vi "Controller.vi"   [LabVIEW 2023]
uses:
  Pulpit/GV_TakePhoto.vi
  GV_exit.vi
  GV_StartStop.vi
  GV_obraz.vi
types:
  T1 = enum16{"Standard", "Buffered", "CRLF", "Immediate"}
  T2 = typedef "IMAQ Image.ctl" = refnum<image>
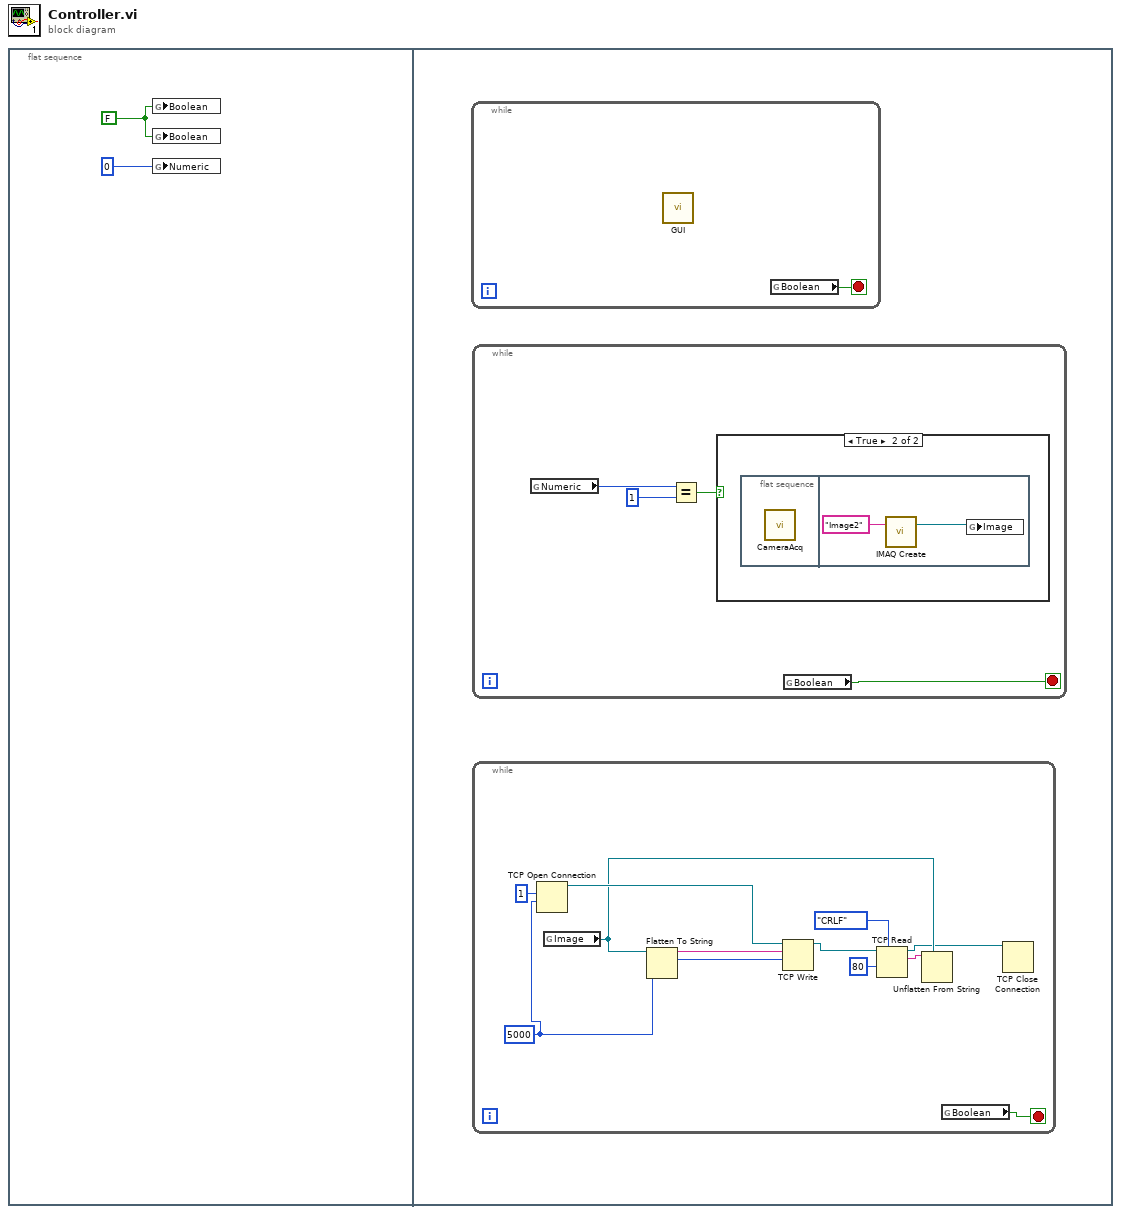
[diagram p0: block diagram]
diagram:
  n1 = flat-sequence {
    frame #0 {
      w1 = FALSE ("Boolean")
      n2 = global write "GV_TakePhoto.vi" "Boolean"(w1) -> ()
      n3 = global write "GV_exit.vi" "Boolean"(w1) -> ()
      n4 = global write "GV_StartStop.vi" "Numeric"(0 ("Numeric")) -> ()
    }
    frame #1 {
      n5 = while {
        stop <- w20 stop-if-true
        n6 = call "GUI.vi"() -> ()  [unwired: 12 in]
        n7 = global read "GV_exit.vi" "Boolean"() -> (w20:bool)
      }
      n8 = while {
        stop <- w15 stop-if-true
        n9 = global read "GV_StartStop.vi" "Numeric"() -> (w14:i32)
        n10 = Equal?(x=w14, y=1) -> (x = y?=w16:bool)
        n11 = case shown="True" w16 {
          frame False {
          }
          frame True {
            n12 = flat-sequence {
              frame #0 {
                n13 = call "CameraAcq.vi"() -> ()  [unwired: 12 in]
              }
              frame #1 {
                n14 = call "IMAQ Create"("Image Name"="Image2") -> ("New Image"=w19:T2)  [unwired: 4 in, 1 out]
                n15 = global write "GV_obraz.vi" "Image"(w19) -> ()
              }
            }
          }
        }
        n16 = global read "GV_exit.vi" "Boolean"() -> (w15:bool)
      }
      n17 = while {
        stop <- w13 stop-if-true
        w6 = 5000 ("timeout ms (25000)")
        n18 = TCP Open Connection(remote port or service name=u16 1, timeout ms (60000)=w6) -> (connection ID=w11:refnum<k5>)  [unwired: 3 in, 1 out]
        n19 = global read "GV_obraz.vi" "Image"() -> (w8:T2)
        n20 = Flatten To String(anything=w8) -> (data string=w12:string)  [unwired: 3 in, 2 out]
        n21 = TCP Write(connection ID=w11, data in=w12, 9:w6) -> (connection ID out=w10:refnum<k5>)  [unwired: 1 in, 2 out]
        n22 = TCP Read(connection ID=w10, 7:T1."CRLF" ("mode (standard)"), 9:80 ("timeout ms (25000)")) -> (connection ID out=w3:refnum<k5>, data out=w9:string)  [unwired: 2 in, 1 out]
        n23 = Unflatten From String(type=w8, binary string=w9) -> ()  [unwired: 3 in, 3 out]
        n24 = global read "GV_exit.vi" "Boolean"() -> (w13:bool)
        n25 = TCP Close Connection(connection ID=w3) -> ()  [unwired: 2 in, 2 out]
      }
    }
  }
